vi "GageTrigLevel.vi"(2 "Voltage Scale":u16(ring)=4, 3 "Trigger Settings":T1={"Source"=1, "Slope"=0, "Coupling"=1, "Trig Input Range"=0, "Level (mV)"=5000, "Trig Depth"=0} {"Trig Input Range" items=["+/- 5 Volts", "+/- 1 Volt"]; "Slope" items=["Positive", "Negative"]; "Level (mV)" min=-5000 max=5000; "Coupling" items=["DC 1 MOhm", "AC 1 MOhm", "DC 50 Ohm", "AC 50 Ohm"]; "Source" items=["Chan A", "Chan B", "External", "Auto"]}) -> (1 "trig level":i16)   [LabVIEW 2022 SP3]
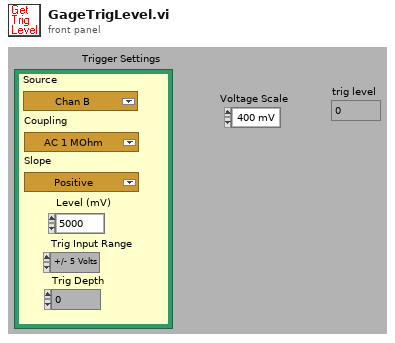
[diagram p1: front panel]
types:
  T1 = cluster{"Source":u16, "Slope":u16, "Coupling":u16, "Trig Input Range":i16, "Level (mV)":i16, "Trig Depth":i32}
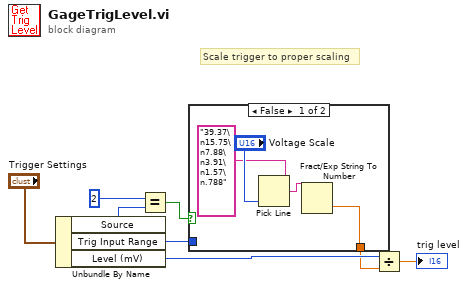
[diagram p0: block diagram]
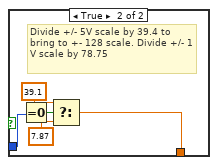
[diagram p2: hidden frame]
diagram:
  # "Scale trigger to proper scaling"
  n1 = Unbundle By Name("Trigger Settings") -> ("Source"=w7:u16, "Trig Input Range"=w3:i16, "Level (mV)"=w8:i16)
  n2 = Equal?(x=2, y=w7) -> (x = y?=w4:bool)
  n3 = case shown="False" w4 {
    tunnel: [w10 w14] -> w5
    tunnel: w3 -> [_ w13]
    frame False {
      n4 = Pick Line(multi-line string="39.37\n15.75\n7.88\n3.91\n1.57\n.788" ("ResourceName"), line index="Voltage Scale") -> (output string=w11:string)  [unwired: 1 out]
      n5 = Fract/Exp String To Number(string=w11) -> (number=w10:dbl)  [unwired: 1 in, 3 out]
    }
    frame True {
      # "Divide +/- 5V scale by 39.4 to bring to +- 128 scale. Divide +/- 1 V scale by 78.75"
      n6 = Equal To 0?(x=w13) -> (x = 0?=w17:bool)
      n7 = Select(t=39.1, s=w17, f=7.87) -> (s? t:f=w14:dbl)
    }
  }
  n8 = Divide(x=w8, y=w5) -> (x/y=→"trig level":dbl)
